vi "Main.vi"() -> ()   [LabVIEW 2019, in "OOP Query Server.lvlib" / "OOP Query Server.lvclass"]
uses:
  OOP Query Server.lvclass
  typeDefs/Server State Data.ctl
  OOP Query Server.lvclass/OOP Query Server.ctl
panel:
  out "error out":errorcluster
  in  "Stop":bool
  in  "Enable Async Mode":bool
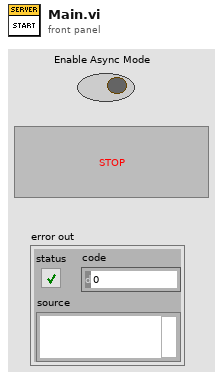
[diagram p1: front panel]
types:
  T1 = typedef "OOP Query Server.lvlib/OOP Query Server.lvclass/Server State Data.ctl" = cluster{"Data":string}
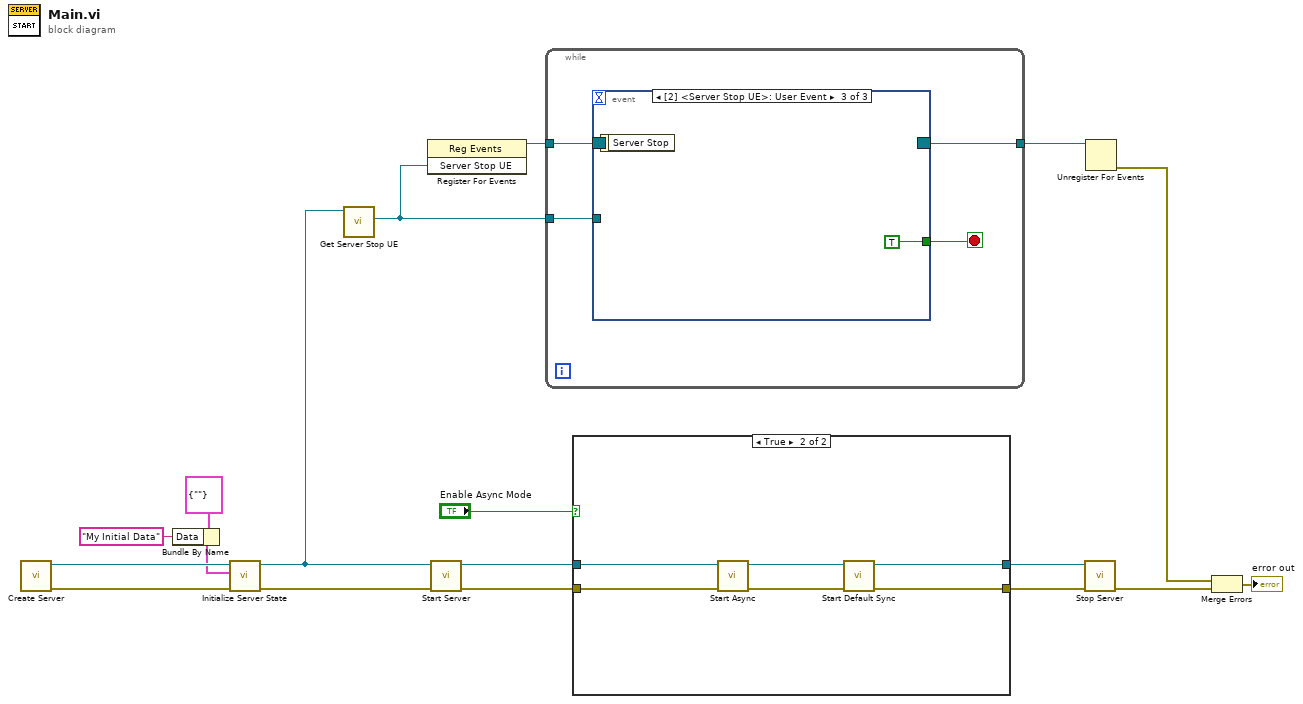
[diagram p0: block diagram]
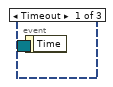
[diagram p2: hidden frame]
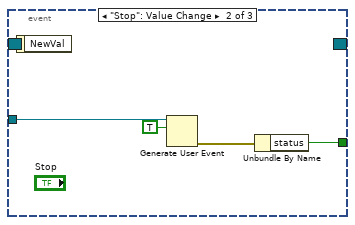
[diagram p3: hidden frame]
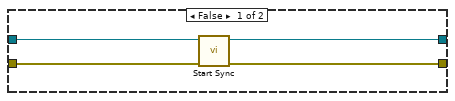
[diagram p4: hidden frame]
diagram:
  n1 = call "Create Server.vi"() -> ("error out"=w7:errorcluster, "gRPC Server out"=w6:refnum<class "OOP Query Server.lvclass">)  [unwired: 10 in]
  n2 = Bundle By Name(cluster=T1 {"Data"=""} ("Initial State"), "Data"="My Initial Data") -> (w2:T1)
  n3 = call "Initialize Server State.vi"("error in (no error)"=w7, "Initial State"=w2, "OOP Query Server in"=w6) -> ("error out"=w5:errorcluster, "OOP Query Server out"=w4:refnum<class "OOP Query Server.lvclass">)  [unwired: 7 in]
  n4 = call "Get Server Stop UE.vi"("OOP Server in"=w4) -> ("Server Stop UE"=w11:refnum<user-event>)  [unwired: 9 in, 1 out]
  n5 = register-events(w11) -> (reference out=w13:refnum<event-registration>)  [unwired: 2 in, 1 out]
  n6 = call "Start Server.vi"("error in (no error)"=w5, "OOP Server in"=w4) -> ("error out"=w18:errorcluster, "gRPC Server out"=w17:refnum<class "OOP Query Server.lvclass">)  [unwired: 8 in]
  n7 = while {
    tunnel: w11 -> [w22]
    tunnel: w13 -> [w21]
    tunnel: [w19] -> w12
    stop <- w20 stop-if-true
    n8 = event shown="[2] <Server Stop UE>: User Event" {
      selector: w21 -> [_ _ _]
      dyn-events: [_ _ _] -> w19
      timeout: _ -> [_ _ _]
      tunnel: w22 -> [_ w26 _]
      tunnel: [_ w23 TRUE] -> w20
      event Timeout {
        n9 = event-data() -> ()  [unwired: 1 in, 1 out]
      }
      event "Stop": Value Change {
        n10 = event-data() -> ()  [unwired: 1 in, 1 out]
        n11 = Generate User Event(user event=w26, event data cluster=TRUE ("event data")) -> (error out=w24:errorcluster)  [unwired: 2 in, 1 out]
        n12 = Unbundle By Name(w24) -> ("status"=w23:bool)
      }
      event User Event {
        n13 = event-data() -> ()  [unwired: 1 in, 1 out]
      }
    }
  }
  n14 = case shown="True" "Enable Async Mode" {
    tunnel: w18 -> [w31 w37]
    tunnel: w17 -> [w30 w36]
    tunnel: [w29 w33] -> w16
    tunnel: [w28 w32] -> w15
    frame False {
      n15 = call "Start Sync.vi"("error in (no error)"=w31, "gRPC Server in"=w30) -> ("error out"=w29:errorcluster, "gRPC Server out"=w28:refnum<class "OOP Query Server.lvclass">)  [unwired: 8 in]
    }
    frame True {
      n16 = call "Start Async.vi"("error in (no error)"=w37, "gRPC Server in"=w36) -> ("error out"=w34:errorcluster, "gRPC Server out"=w35:refnum<class "OOP Query Server.lvclass">)  [unwired: 8 in]
      n17 = call "Start Default Sync.vi"("error in (no error)"=w34, "gRPC Server in"=w35) -> ("error out"=w33:errorcluster, "gRPC Server out"=w32:refnum<class "OOP Query Server.lvclass">)  [unwired: 8 in]
    }
  }
  n18 = call "Stop Server.vi"("error in (no error)"=w16, "gRPC Server in"=w15) -> ("error out"=w10:errorcluster)  [unwired: 9 in]
  n19 = Unregister For Events(event registration refnum=w12) -> (error out=w9:errorcluster)  [unwired: 1 in]
  n20 = Merge Errors(w9, w10) -> (→"error out":errorcluster)
